vi "Digital Read Port Test.vi"() -> ()   [LabVIEW 2011]
uses:
  Private/Type Defs/Chipkit Configuration.ctl
  Private/Type Defs/Board Type.ctl
  LabVIEW Interface for ChipKit.lvlib
panel:
  in  "ChipKit Configuration":T1
  out "size(s)":i32
  out "Digital Port":bool[](array[boolean])
  in  "Stop Button":bool
  in  "DIO Pins":u8[](array[numeric])=[2, 3, 4, 5, 23, 25, 27, 29, 13, 12, 11]
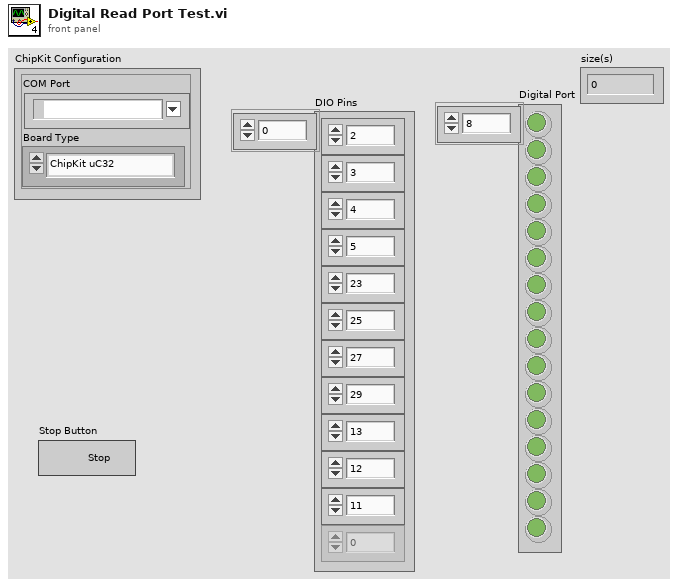
[diagram p1: front panel]
types:
  T1 = typedef "LabVIEW Interface for ChipKit.lvlib/Chipkit Configuration.ctl" = cluster{"COM Port":refnum<visa-resource-name>, "Board Type":T2}
  T2 = typedef "LabVIEW Interface for ChipKit.lvlib/Board Type.ctl" = enum16{"ChipKit uC32", "ChipKit Uno32", "ChipKit Max32"}
  T3 = typedef "LabVIEW Interface for ChipKit.lvlib/Chipkit Resource.ctl" = cluster{"COM Port":refnum<visa-resource-name>, "Board Type":T2, "Connection Type":T4, "Baud Rate (115200)":u32, "Bytes Per Packet (15)":u32, "DI Port Num Pins":i32, "DO Port Num Pins":i32}
  T4 = typedef "LabVIEW Interface for ChipKit.lvlib/Connection Type.ctl" = enum8{"USB / Serial", "XBEE", "BlueSmirf (Bluetooth)"}
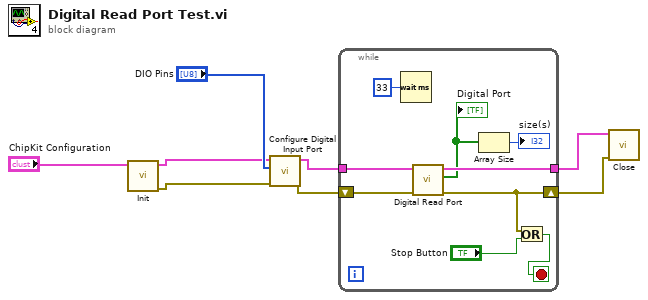
[diagram p0: block diagram]
diagram:
  n1 = call "Init.vi"("ChipKit Configuration"="ChipKit Configuration") -> ("Error Out"=w1:errorcluster, "ChipKit Configuration"=w2:T3)  [unwired: 9 in]
  n2 = call "Configure Digital Input Port.vi"("Error In"=w1, "DI Pins"="DIO Pins", "ChipKit Resource"=w2) -> ("Error Out"=w5:errorcluster, "ChipKit Resource"=w7:T3)  [unwired: 7 in]
  n3 = while {
    tunnel: w7 -> [w17]
    tunnel: [w16] -> w6
    shift-right: [w12] -> w4
    shift-left: w5 -> [w15]
    stop <- w13 stop-if-true
    n4 = Wait (ms)(milliseconds to wait=u32 33) -> ()  [unwired: 1 out]
    n5 = call "Digital Read Port.vi"("Error In"=w15, "ChipKit Resource"=w17) -> ("Error Out"=w12:errorcluster, "Digital Port"=w11:bool[], "ChipKit Resource"=w16:T3)  [unwired: 7 in]
    "Digital Port" <- w11
    n6 = Array Size(array=w11) -> (size(s)=→"size(s)":i32)
    n7 = Or(x=w12, y="Stop Button") -> (x .or. y?=w13:bool)
  }
  n8 = call "Close.vi"("Error In"=w4, "ChipKit Configuration"=w6) -> ()  [unwired: 9 in, 1 out]
